vi "ClassBannerEditor_Facade.vi"(0 "Data In":T6, 2 "Display State In":T2={"CurrentIcon"={"Icon Text"="Default", "RectangleColors"={"Border"=16777215, "Background"=0}, "FontSettings"={"Size"=9, "Capitalize text"=TRUE, "TextColor"=0}}}, 3 "Container State":T5) -> (6 "Data Out":T6, 7 "Display State Out":T2={"CurrentIcon"={"Icon Text"="Default", "RectangleColors"={"Border"=16777215, "Background"=0}, "FontSettings"={"Size"=9, "Capitalize text"=TRUE, "TextColor"=0}}}, 8 "Action":T1)   [LabVIEW 2014, in "ClassBannerEditor.xctl"]
uses:
  ClassBannerEditor.xctl
  ClassBannerEditor_Data.ctl
  <vilib>/LabVIEW Icon API/lv_icon/Classes/Icon/Icon.lvclass
  <vilib>/_xctls/Container State.ctl
  ClassBannerEditor_State.ctl
  <vilib>/LabVIEW Icon API/API_Rectangle Colors.ctl
  ClassBannerEditor_FontSettings.ctl
  <vilib>/_xctls/Action.ctl
  <vilib>/LabVIEW Icon API/lv_icon/Classes/Icon Framework/Icon Framework.lvclass
  <vilib>/_xctls/XControlSupport.lvlib
  ClassIconTools/ClassIconTools.lvlib
  <vilib>/LabVIEW Icon API/LabVIEW Icon API.lvlib
panel:
  in  "Capital":bool
  in  "Text Size":u8=9
  in  "Icon Text":string="Default"
  in  "Border Color":u32(colorbox)
  in  "Fill Color":u32(colorbox)=16448250
  in  "Text Color":u32(colorbox)
  out "Icon":picture caption="Preview"
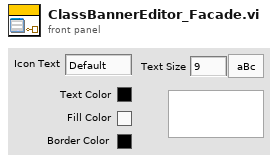
[diagram p1: front panel]
types:
  T1 = typedef "XControlSupport.lvlib/Action.ctl" = cluster{"Data Changed?":bool, "State Changed?":bool, "Action Name":string}
  T2 = typedef "ClassBannerEditor.xctl/ClassBannerEditor_State.ctl" = cluster{"CurrentIcon":cluster{"Icon Text":string, "RectangleColors":T3, "FontSettings":T4}}
  T3 = typedef "LabVIEW Icon API.lvlib/API_Rectangle Colors.ctl" = cluster{"Border":u32, "Background":u32}
  T4 = typedef "ClassBannerEditor.xctl/ClassBannerEditor_FontSettings.ctl" = cluster{"Size":u8, "Capitalize text":bool, "TextColor":u32}
  T5 = typedef "XControlSupport.lvlib/Container State.ctl" = cluster{"Indicator?":bool, "Run Mode?":bool, " Refnum":refnum<vi>}
  T6 = typedef "ClassBannerEditor.xctl/ClassBannerEditor_Data.ctl" = refnum<class "Icon.lvclass">
  T7 = typedef "BodyText.ctl" = cluster{"Line 1 text":string, "Line 2 text":string, "Line 3 text":string, "Line 4 text":string, "Line 1 color":u32, "Line 2 color":u32, "Line 3 color":u32, "Line 4 color":u32, "Body Text Spec":cluster{"Font":T8, "Alignment":T9, "Size":u8}, "Center text vertically":bool, "Capitalize Text":bool}
  T8 = typedef "Font.ctl" = string
  T9 = typedef "Alignment.ctl" = u16
  T10 = typedef "imagedata.ctl" = cluster{"image type":i32, "image depth":i32, "image":u8[], "mask":u8[], "colors":u32[], "Rectangle":cluster{"left":i16, "top":i16, "right":i16, "bottom":i16}}
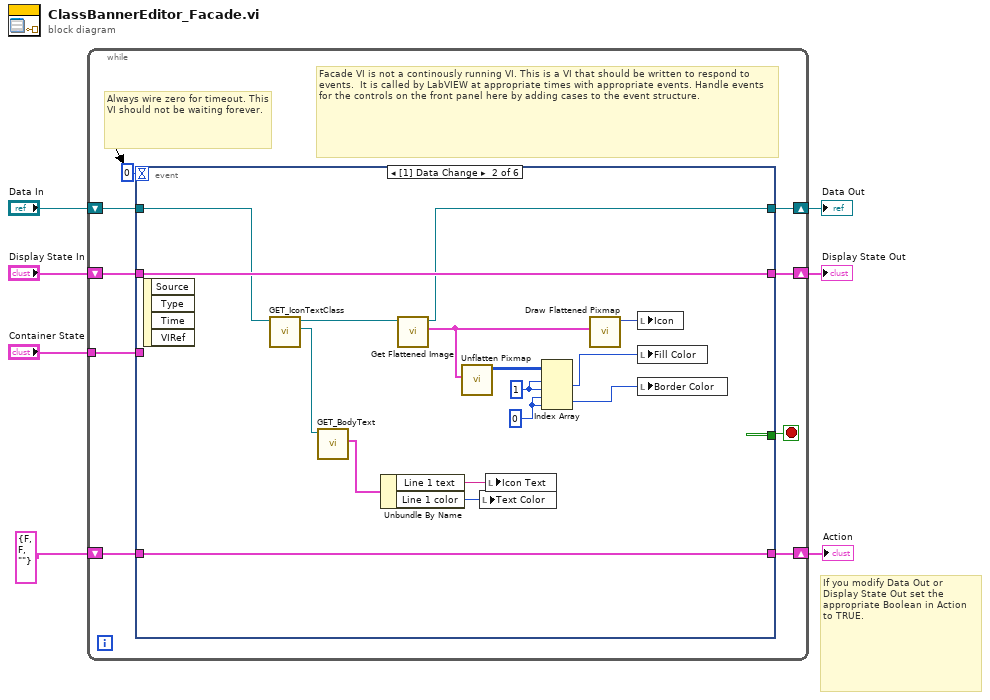
[diagram p0: block diagram]
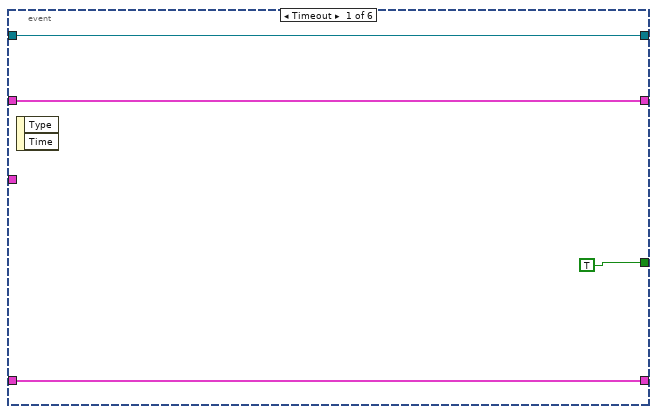
[diagram p2: hidden frame]
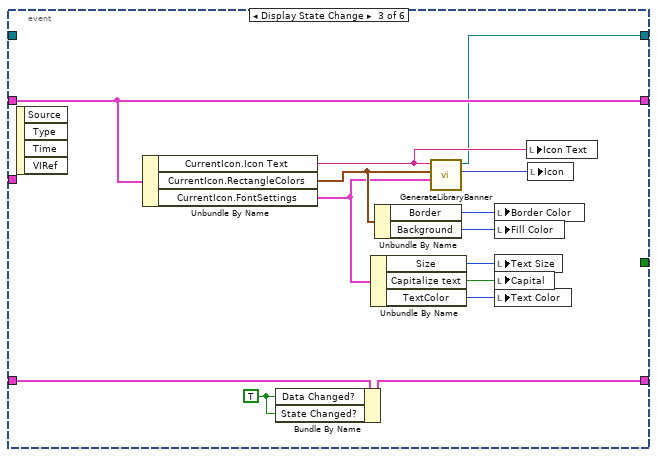
[diagram p3: hidden frame]
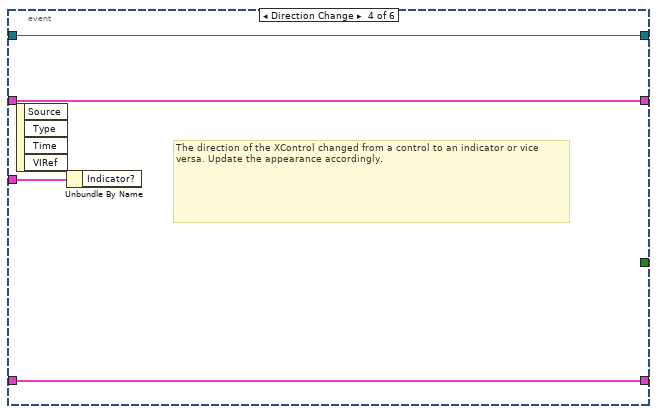
[diagram p4: hidden frame]
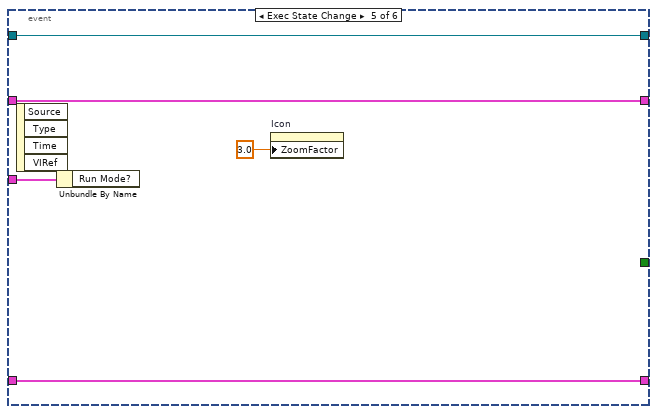
[diagram p5: hidden frame]
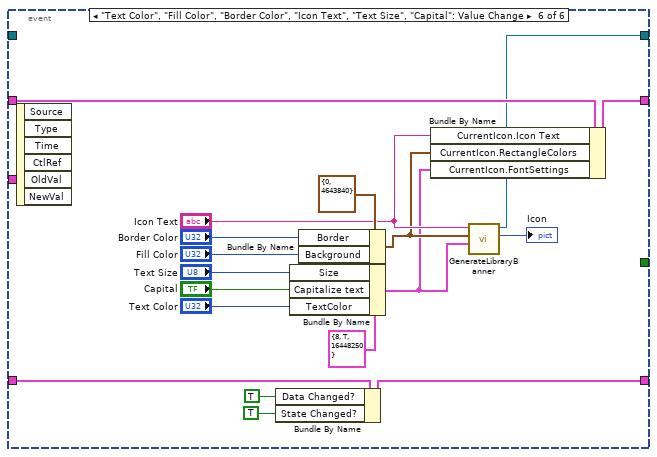
[diagram p6: hidden frame]
diagram:
  # "If you modify Data Out or\nDisplay State Out set the\nappropriate Boolean in Action\nto TRUE."
  n1 = while {
    shift-right: [w15] -> w4
    shift-left: "Display State In" -> [w16]
    tunnel: "Container State" -> [w12]
    shift-right: [w10] -> w7
    shift-left: "Data In" -> [w11]
    shift-right: [w8] -> w2
    shift-left: T1 {"Data Changed?"=FALSE, "State Changed?"=FALSE, "Action Name"=""} ("Action") -> [w9]
    stop <- w14 stop-if-true
    # "Facade VI is not a continously running VI. This is a VI that should be written to respond to events.  It is called by LabVIEW at appropriate times with appropriate events. Handle events for the controls on the front panel here by adding cases to the event structure."
    # "Always wire zero for timeout. This\nVI should not be waiting forever."
    n2 = event shown="[1] Data Change" {
      selector: _ -> [_ _ _ _ _ _]
      dyn-events: _ -> [_ _ _ _ _ _]
      timeout: 0 -> [_ _ _ _ _ _]
      tunnel: w16 -> [w18 w36 w48 w53 w56 w77]
      tunnel: [w18 w36 w48 w53 w56 w63] -> w15
      tunnel: [TRUE _ _ _ _ _] -> w14
      tunnel: w12 -> [_ _ _ w54 w59 _]
      tunnel: w11 -> [w17 w32 _ w52 w57 _]
      tunnel: [w17 w34 w39 w52 w57 w73] -> w10
      tunnel: [w19 w35 w38 w51 w58 w71] -> w8
      tunnel: w9 -> [w19 w35 w50 w51 w58 w76]
      event Timeout {
        n3 = event-data() -> ()  [unwired: 1 in, 2 out]
      }
      event Data Change {
        w23 = 0 ("index (col)")
        w25 = 1 ("index (row)")
        n4 = event-data() -> ()  [unwired: 1 in, 4 out]
        n5 = call-dynamic "GET_IconTextClass.vi"("Icon.lvclass in"=w32) -> ("Icon Framework.lvclass"=w30:refnum<class "Icon Framework.lvclass">, "Icon.lvclass out"=w31:T6)  [unwired: 8 in, 1 out]
        n6 = call-dynamic "GET_BodyText.vi"("Icon Framework.lvclass in"=w30) -> ("Body Text"=w29:T7)  [unwired: 7 in, 3 out]
        n7 = Unbundle By Name(w29) -> ("Line 1 text"=w28:string, "Line 1 color"=w27:u32)
        n8 = call <vilib>:"Get Flattened Image.vi"("lv_icon.lvlib:Icon.lvclass in"=w31) -> ("Color Image"=w24:T10, "lv_icon.lvlib:Icon.lvclass out"=w34:T6)  [unwired: 7 in, 2 out]
        n9 = call <vilib>:"Unflatten Pixmap.vi"("image data"=w24) -> ("24-bit pixmap"=w26:u32[][])  [unwired: 4 in, 6 out]
        n10 = local write "Text Color"(w27) -> ()
        n11 = local write "Icon Text"(w28) -> ()
        n12 = Index Array(array=w26, index (row) #1=w25, index (col) #1=w25, index (row) #2=w23, index (col) #2=w23) -> (element #1=w22:u32, element #2=w21:u32)
        n13 = call <vilib>:"Draw Flattened Pixmap.vi"("image data"=w24) -> ("new picture"=w33:picture)  [unwired: 8 in]
        n14 = local write "Icon"(w33) -> ()
        n15 = local write "Fill Color"(w22) -> ()
        n16 = local write "Border Color"(w21) -> ()
      }
      event Display State Change {
        w37 = TRUE ("Data Changed?")
        n17 = event-data() -> ()  [unwired: 1 in, 4 out]
        n18 = Unbundle By Name(w48) -> ("CurrentIcon.Icon Text"=w47:string, "CurrentIcon.RectangleColors"=w46:T3, "CurrentIcon.FontSettings"=w43:T4)
        n19 = Bundle By Name(cluster=w50, "Data Changed?"=w37, "State Changed?"=w37) -> (w38:T1)
        n20 = Unbundle By Name(w43) -> ("Size"=w42:u8, "Capitalize text"=w41:bool, "TextColor"=w40:u32)
        n21 = Unbundle By Name(w46) -> ("Border"=w45:u32, "Background"=w44:u32)
        n22 = call "GenerateLibraryBanner.vi"("Text settings"=w43, "Rectangle colors (black, white)"=w46, "Text"=w47) -> ("Picture"=w49:picture, "Icon.lvlclass out"=w39:refnum<class "Icon.lvclass">)  [unwired: 6 in, 1 out]
        n23 = local write "Border Color"(w45) -> ()
        n24 = local write "Fill Color"(w44) -> ()
        n25 = local write "Text Size"(w42) -> ()
        n26 = local write "Capital"(w41) -> ()
        n27 = local write "Text Color"(w40) -> ()
        n28 = local write "Icon Text"(w47) -> ()
        n29 = local write "Icon"(w49) -> ()
      }
      event Direction Change {
        # "The direction of the XControl changed from a control to an indicator or vice versa. Update the appearance accordingly."
        n30 = event-data() -> ()  [unwired: 1 in, 4 out]
        n31 = Unbundle By Name(w54) -> ()  [unwired: 1 out]
      }
      event Exec State Change {
        n32 = event-data() -> ()  [unwired: 1 in, 4 out]
        n33 = Unbundle By Name(w59) -> ()  [unwired: 1 out]
        n34 = property on="Icon" class="Pict"("ZoomFactor"=sgl 3.0 ("Zoom Factor")) -> ()  [unwired: 2 in, 2 out]
      }
      event "Text Color", "Fill Color", "Border Color", "Icon Text", "Text Size", "Capital": Value Change {
        n35 = event-data() -> ()  [unwired: 1 in, 6 out]
        n36 = Bundle By Name(cluster=w76, "Data Changed?"=TRUE, "State Changed?"=TRUE) -> (w71:T1)
        n37 = Bundle By Name(cluster=T4 {"Size"=8, "Capitalize text"=TRUE, "TextColor"=16448250} ("Text settings"), "Size"="Text Size", "Capitalize text"="Capital", "TextColor"="Text Color") -> (w60:T4)
        n38 = Bundle By Name(cluster=T3 {"Border"=0, "Background"=4643840} ("Rectangle colors (black, white)"), "Border"="Border Color", "Background"="Fill Color") -> (w61:T3)
        n39 = Bundle By Name(cluster=w77, "CurrentIcon.Icon Text"="Icon Text", "CurrentIcon.RectangleColors"=w61, "CurrentIcon.FontSettings"=w60) -> (w63:T2)
        n40 = call "GenerateLibraryBanner.vi"("Text settings"=w60, "Rectangle colors (black, white)"=w61, "Text"="Icon Text") -> ("Picture"=→"Icon":picture, "Icon.lvlclass out"=w73:refnum<class "Icon.lvclass">)  [unwired: 6 in, 1 out]
      }
    }
  }
  "Display State Out" <- w4
  "Data Out" <- w7
  "Action" <- w2
